vi "Memory.Pointer.Advanced Copy.vi"(0 "src Pointer in":refnum<class "Memory.Pointer.lvclass">, 1 "dst width":u64 format="%d bytes", 2 "src width":u64 format="%d bytes", 5 "dst Pointer in":refnum<class "Memory.Pointer.lvclass">, 7 "src offset (0)":u64 format="%d bytes", 9 "dst offset (0)":u64 format="%d bytes", 11 "error in (no error)":errorcluster, 12 "src byte order (little-endian)":enum16{"big-endian", "little-endian"}(ring)=enum."little-endian", 13 "dst byte order (little-endian)":enum16{"big-endian", "little-endian"}(ring)=enum."little-endian", 14 "clear dst bytes? (T)":bool=TRUE) -> (4 "src Pointer out":refnum<class "Memory.Pointer.lvclass">, 6 "dst Pointer out":refnum<class "Memory.Pointer.lvclass">, 15 "error out":errorcluster)   [LabVIEW 2016, in "Memory Manager.lvlib" / "Memory.Pointer.lvclass"]
doc: "Moves bytes of data from the <b>src pointer</b> at <b>src offset</b> to the <b>dst pointer</b> at <b>dst offset</b> using the <b>byte order</b> specified. <b>src width</b> and <b>dst width</b> are used to determine how many bytes to move, as well as where the bytes should be read from/written to in memory. For example, to type cast a DBL to a U16, src width would be 8 bytes and dst width would be 2 bytes.\n\nThe optional argument <b>clear dst bytes</b> will clear the subset of bytes within <b>dst pointer</b> before moving data from the <b>src pointer</b>. This is required when type casting from a smaller type to a larger type, as the larger type may have non-zero bytes that will not get overwritten. This argument can be set the FALSE when casting larger types down to smaller types.\n\n<b>Note:</b> This VI is <b>safe</b>, meaning it performs null pointer and bounds checks to prevent invalid memory access."
uses:
  Memory.Pointer.lvclass
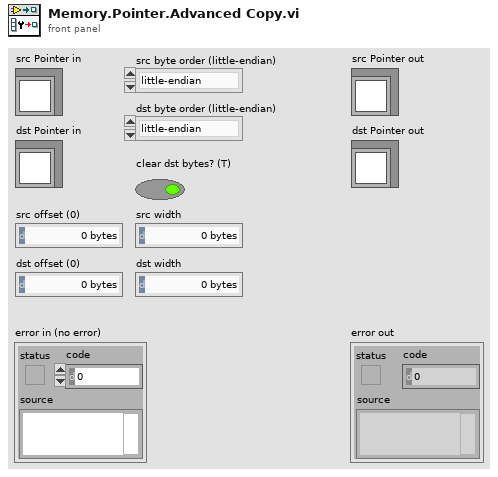
[diagram p1: front panel]
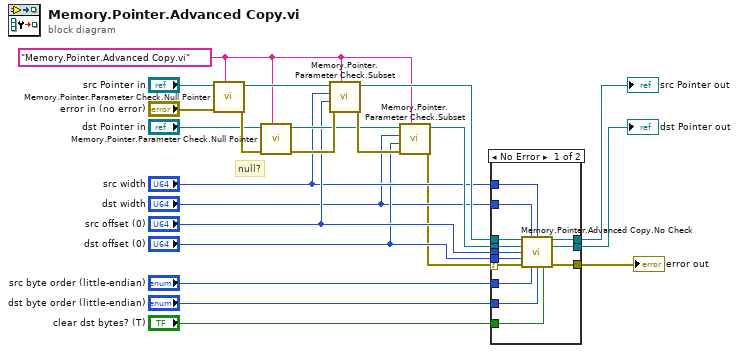
[diagram p0: block diagram]
diagram:
  w8 = "Memory.Pointer.Advanced Copy.vi" ("source vi name")
  # "null?"
  n1 = call "Memory.Pointer.Parameter Check.Null Pointer.vi"("source vi name"=w8, "error in (no error)"="error in (no error)", "Pointer in"="src Pointer in") -> ("error out"=w21:errorcluster, "Pointer out"=w14:refnum<class "Memory.Pointer.lvclass">)  [unwired: 7 in]
  n2 = call "Memory.Pointer.Parameter Check.Null Pointer.vi"("source vi name"=w8, "error in (no error)"=w21, "Pointer in"="dst Pointer in") -> ("error out"=w20:errorcluster, "Pointer out"=w13:refnum<class "Memory.Pointer.lvclass">)  [unwired: 7 in]
  n3 = call "Memory.Pointer.Parameter Check.Subset.vi"("source vi name"=w8, "error in (no error)"=w20, "offset (0)"="src offset (0)", "length"="src width", "Pointer in"=w14) -> ("error out"=w22:errorcluster, "Pointer out"=w11:refnum<class "Memory.Pointer.lvclass">)  [unwired: 3 in, 2 out]
  n4 = call "Memory.Pointer.Parameter Check.Subset.vi"("source vi name"=w8, "error in (no error)"=w22, "offset (0)"="dst offset (0)", "length"="dst width", "Pointer in"=w13) -> ("error out"=w3:errorcluster, "Pointer out"=w12:refnum<class "Memory.Pointer.lvclass">)  [unwired: 3 in, 2 out]
  n5 = case shown="No Error" w3 {
    selector: w3 -> [w26 w36]
    tunnel: [w35 w36] -> w18
    tunnel: "clear dst bytes? (T)" -> [w25 _]
    tunnel: w12 -> [w34 w37]
    tunnel: w11 -> [w33 w38]
    tunnel: [w32 w37] -> w10
    tunnel: [w31 w38] -> w9
    tunnel: "src offset (0)" -> [w30 _]
    tunnel: "src width" -> [w29 _]
    tunnel: "dst offset (0)" -> [w28 _]
    tunnel: "dst width" -> [w27 _]
    tunnel: "src byte order (little-endian)" -> [w24 _]
    tunnel: "dst byte order (little-endian)" -> [w23 _]
    frame No Error {
      n6 = call "Memory.Pointer.Advanced Copy.No Check.vi"("src Pointer in"=w33, "dst width"=w27, "src width"=w29, "dst Pointer in"=w34, "src offset (0)"=w30, "dst offset (0)"=w28, "error in (no error)"=w26, "src byte order (little-endian)"=w24, "dst byte order (little-endian)"=w23, "clear dst bytes? (T)"=w25) -> ("src Pointer out"=w31:refnum<class "Memory.Pointer.lvclass">, "dst Pointer out"=w32:refnum<class "Memory.Pointer.lvclass">, "error out"=w35:errorcluster)  [unwired: 3 in]
    }
    frame Error {
    }
  }
  "error out" <- w18
  "src Pointer out" <- w9
  "dst Pointer out" <- w10
